vi "Create.vi"(8 "error in (no error)":errorcluster, 11 "Timeout":i32) -> (0 "error out":errorcluster, 3 "Stop DAQ Timeout Msg out":refnum<class "Stop DAQ Timeout Msg.lvclass">)   [LabVIEW 2012, in "Configuration Grandmaster.lvlib" / "Stop DAQ Timeout Msg.lvclass"]
uses:
  Stop DAQ Timeout Msg.lvclass
  Stop DAQ Timeout Msg.lvclass/Stop DAQ Timeout Msg.ctl
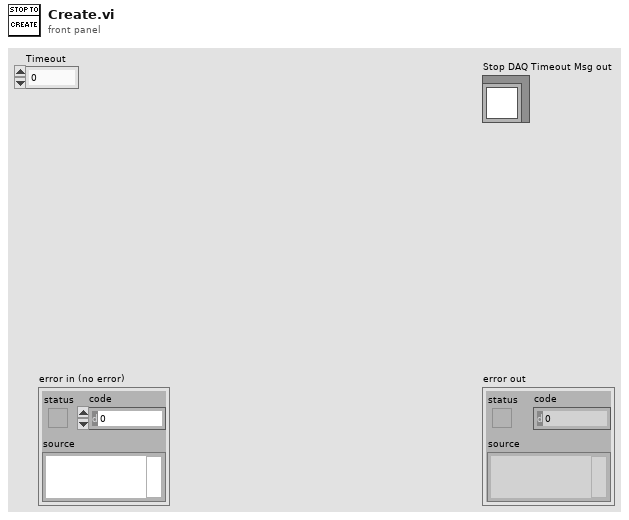
[diagram p1: front panel]
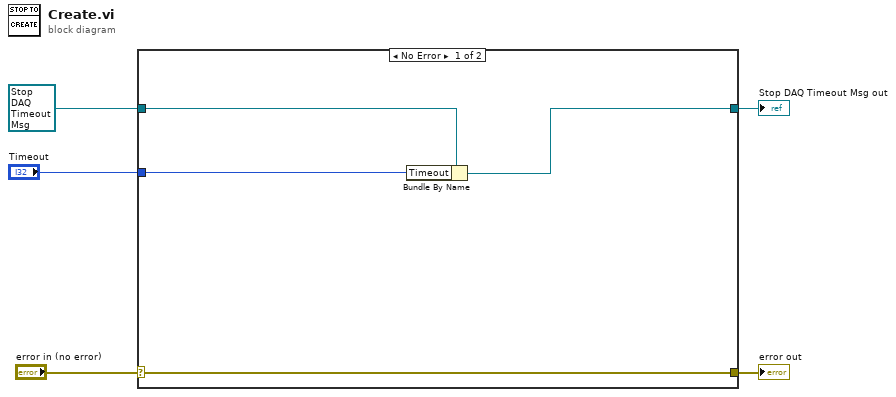
[diagram p0: block diagram]
diagram:
  n1 = case shown="No Error" "error in (no error)" {
    selector: "error in (no error)" -> [w9 w11]
    tunnel: [w9 w11] -> w4
    tunnel: [w7 w10] -> w2
    tunnel: refnum<class "Stop DAQ Timeout Msg.lvclass"> refnum ("Stop DAQ Timeout Msg in") -> [w8 w10]
    tunnel: "Timeout" -> [w6 _]
    frame No Error {
      n2 = Bundle By Name(cluster=w8, "Timeout"=w6) -> (w7:refnum<class "Stop DAQ Timeout Msg.lvclass">)
    }
    frame Error {
    }
  }
  "error out" <- w4
  "Stop DAQ Timeout Msg out" <- w2
